vi "FP_VI Pane Show Hide Scrollbars.vi"(8 "Error":errorcluster, 9 "Scrollbar Settings":T1, 10 "Pane Index":i32, 11 "VI":refnum<vi>) -> (0 "Error Out":errorcluster, 3 "VI Out":refnum<vi>)   [LabVIEW 2023]
uses:
  TypeDefs_Utility/Cluster_FP_Scroll Bars Hide Show.ctl
  TypeDefs_Utility/ENUM_FP_Show-Hide Select.ctl
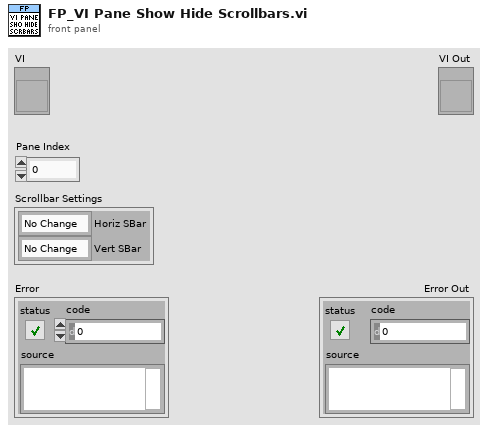
[diagram p1: front panel]
types:
  T1 = typedef "Cluster_FP_Scroll Bars Hide Show.ctl" = cluster{"Horiz SBar":T2, "Vert SBar":T2}
  T2 = typedef "ENUM_FP_Show-Hide Select.ctl" = enum16{"No Change", "Hide", "Show"}
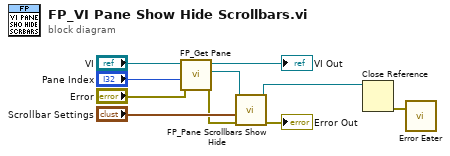
[diagram p0: block diagram]
diagram:
  n1 = call "FP_Get Pane.vi"("Error"="Error", "Pane Index"="Pane Index", "VI"="VI") -> ("Error Out"=w5:errorcluster, "Pane Refnum Out"=w7:refnum<vi>, "VI Out"=→"VI Out":refnum<vi>)  [unwired: 6 in]
  n2 = call "FP_Pane Scrollbars Show Hide.vi"("Error"=w5, "Scrollbar Settings"="Scrollbar Settings", "Pane"=w7) -> ("Error Out"=→"Error Out":errorcluster, "Pane Out"=w3:refnum<vi>)  [unwired: 7 in]
  n3 = Close Reference(reference=w3) -> (error out=w2:errorcluster)  [unwired: 1 in]
  n4 = call "Error Eater.vi"("error in (no error)"=w2) -> ()  [unwired: 2 in]
